vi "test Configure SLSC Switch Custom Device from Switches JSON.vi"(8 "error in (no error)":errorcluster, 11 "TestCase in":refnum<class "NI-SWITCH Scripting Unit Tests.lvclass">) -> (0 "error out":errorcluster, 3 "TestCase out":refnum<class "NI-SWITCH Scripting Unit Tests.lvclass">)   [LabVIEW 2017, in "NI-SWITCH Scripting Unit Tests.lvclass"]
uses:
  NI-SWITCH Scripting Unit Tests.lvclass
  <vilib>/addons/_JKI Toolkits/VI Tester/TestCase.llb/TestCase.lvclass
  NI-SWITCH Scripting.lvlib
  Shared/Endpoint Configuration Enum.ctl
  Shared/NI-SWITCH Shared.lvlib
  Shared/Endpoint Configuration Cluster.ctl
  Custom Device/Find All SLSC Switch Custom Devices.vi
  Shared/Routing and Faulting Hardware API/Routing and Faulting Hardware API.lvlib
  C:/Program Files (x86)/National Instruments/LabVIEW 2017/vi.lib/addons/_JKI Toolkits/VI Tester/TestCase.llb/TestCase.lvclass
panel:
  in  "Save?":bool
  out "Output Filename":string
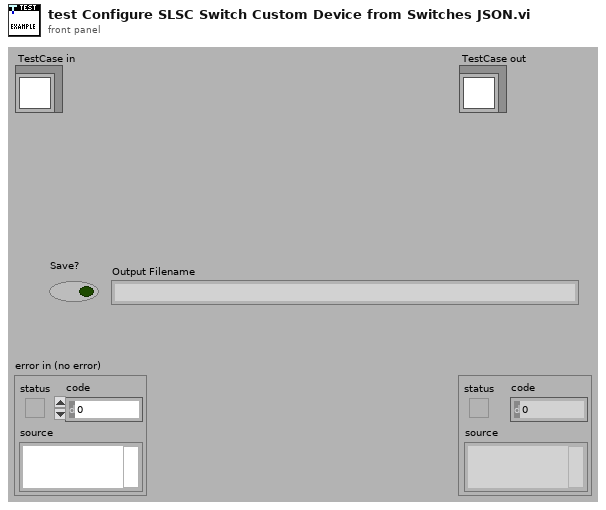
[diagram p1: front panel]
types:
  T1 = typedef "NI-SWITCH Shared.lvlib/Endpoint Configuration Cluster.ctl" = cluster{"Endpoint":string, "Configuration":T2}
  T2 = typedef "NI-SWITCH Shared.lvlib/Endpoint Configuration Enum.ctl" = enum16{"Load", "Source", "Configuration"}
  T3 = typedef "Custom Device API.lvlib/Custom Device Item Ref.ctl" = u64
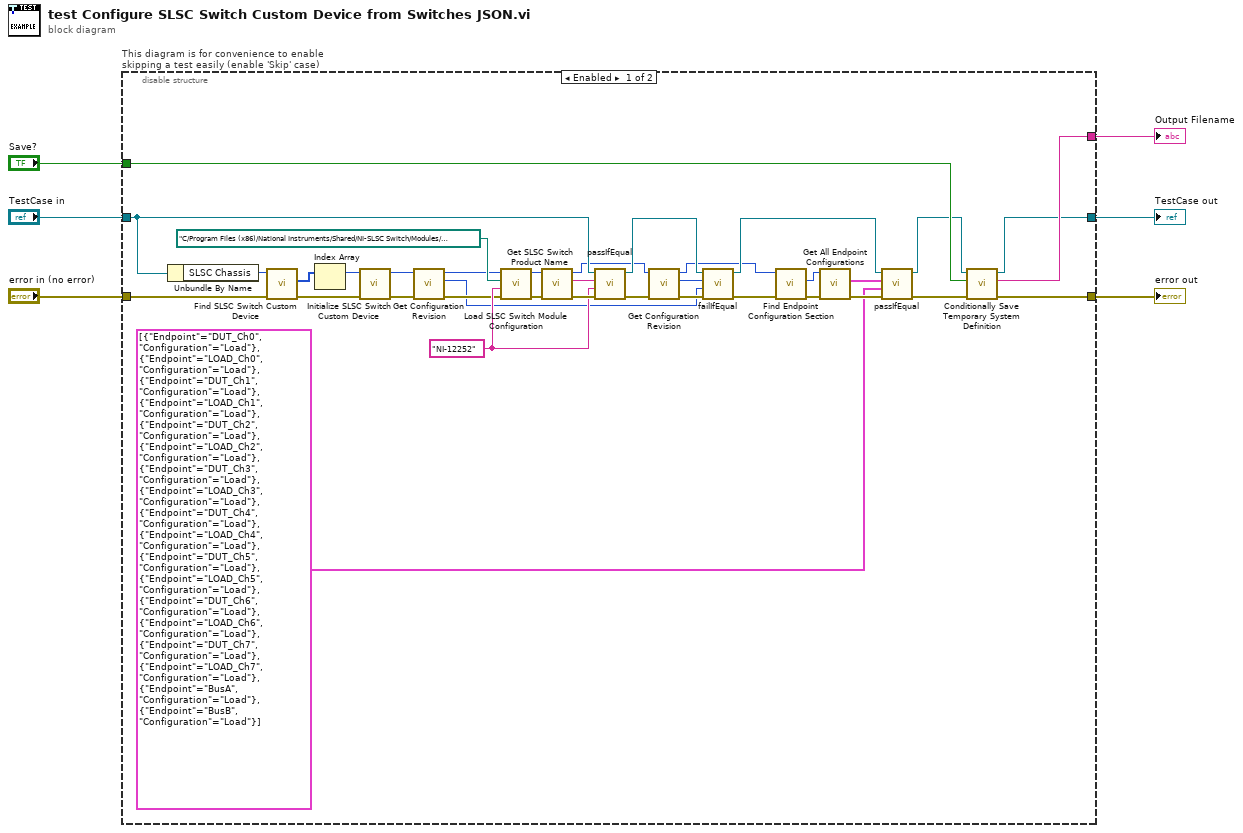
[diagram p0: block diagram]
diagram:
  n1 = disable-structure "This diagram is for convenience to enable skipping a test easily (enable 'Skip' case)" shown="Enabled" {
    disable-tunnel: "TestCase in" -> [w32 w46]
    disable-tunnel: [w40 w44] -> w3
    disable-tunnel: [w41 w45] -> w5
    disable-tunnel: "error in (no error)" -> [w36 w43]
    disable-tunnel: [w42 _] -> w2
    disable-tunnel: "Save?" -> [w39 _]
    frame Enabled {
      w20 = "NI-12252" ("Model")
      n2 = Unbundle By Name(w32) -> ("SLSC Chassis"=w37:u64)
      n3 = call-poly "Find SLSC Switch Custom Device.vi"("error in"=w36, "slsc chassis in"=w37) -> ("error out"=w34:errorcluster, "slsc switch custom devices"=w38:T3[])  [unwired: 7 in, 1 out]
      n4 = Index Array(array=w38) -> (element=w35:T3)  [unwired: 1 in]
      n5 = call "Initialize SLSC Switch Custom Device.vi"("error in"=w34, "slsc switch custom device in"=w35) -> ("error out"=w19:errorcluster, "slsc switch custom device out"=w17:T3)  [unwired: 7 in, 1 out]
      n6 = call "Get Configuration Revision.vi"("error in (no error)"=w19, "Hardware Ref in"=w17) -> ("error out"=w18:errorcluster, "Configuration Revision"=w10:u32, "Hardware Ref out"=w16:T3)  [unwired: 6 in, 1 out]
      n7 = call "Load SLSC Switch Module Configuration.vi"("error in"=w18, "product name"=w20, "switches json file"=path "C:/Program Files (x86)/National Instruments/Shared/NI-SLSC Switch/Modules/SLSC-12252-switches.json" ("switches JSON file"), "slsc switch custom device in"=w16) -> ("error out"=w21:errorcluster, "slsc switch custom device out"=w31:T3)  [unwired: 6 in]
      n8 = call "Get SLSC Switch Product Name.vi"("error in"=w21, "slsc switch custom device in"=w31) -> ("error out"=w30:errorcluster, "product name"=w29:string, "slsc switch custom device out"=w8:T3)  [unwired: 7 in]
      n9 = call-dynamic "passIfEqual.vi"("error in (no error)"=w30, "y"=w20, "x"=w29, "TestCase in"=w32) -> ("error out"=w13:errorcluster, "TestCase out"=w15:refnum<class "NI-SWITCH Scripting Unit Tests.lvclass">)  [unwired: 6 in]
      n10 = call "Get Configuration Revision.vi"("error in (no error)"=w13, "Hardware Ref in"=w8) -> ("error out"=w12:errorcluster, "Configuration Revision"=w11:u32, "Hardware Ref out"=w7:T3)  [unwired: 6 in, 1 out]
      n11 = call-dynamic "failIfEqual.vi"("error in (no error)"=w12, "y"=w10, "x"=w11, "TestCase in"=w15) -> ("error out"=w9:errorcluster, "TestCase out"=w14:refnum<class "NI-SWITCH Scripting Unit Tests.lvclass">)  [unwired: 6 in]
      n12 = call "Find Endpoint Configuration Section.vi"("error in"=w9, "slsc switch custom device in"=w7) -> ("error out"=w25:errorcluster, "endpoint configuration"=w24:T3)  [unwired: 7 in, 1 out]
      n13 = call "Get All Endpoint Configurations.vi"("error in"=w25, "endpoint configuration in"=w24) -> ("error out"=w28:errorcluster, "endpoint configurations"=w22:T1[])  [unwired: 7 in, 1 out]
      n14 = call-dynamic "passIfEqual.vi"("error in (no error)"=w28, "y"=T1[] [{"Endpoint"="DUT_Ch0", "Configuration"=enum."Load"}, {"Endpoint"="LOAD_Ch0", "Configuration"=enum."Load"}, {"Endpoint"="DUT_Ch1", "Configuration"=enum."Load"}, {"Endpoint"="LOAD_Ch1", "Configuration"=enum."Load"}, {"Endpoint"="DUT_Ch2", "Configuration"=enum."Load"}, {"Endpoint"="LOAD_Ch2", "Configuration"=enum."Load"}, {"Endpoint"="DUT_Ch3", "Configuration"=enum."Load"}, {"Endpoint"="LOAD_Ch3", "Configuration"=enum."Load"}, {"Endpoint"="DUT_Ch4", "Configuration"=enum."Load"}, {"Endpoint"="LOAD_Ch4", "Configuration"=enum."Load"}, {"Endpoint"="DUT_Ch5", "Configuration"=enum."Load"}, {"Endpoint"="LOAD_Ch5", "Configuration"=enum."Load"}, {"Endpoint"="DUT_Ch6", "Configuration"=enum."Load"}, {"Endpoint"="LOAD_Ch6", "Configuration"=enum."Load"}, {"Endpoint"="DUT_Ch7", "Configuration"=enum."Load"}, {"Endpoint"="LOAD_Ch7", "Configuration"=enum."Load"}, {"Endpoint"="BusA", "Configuration"=enum."Load"}, {"Endpoint"="BusB", "Configuration"=enum."Load"}] ("All Endpoint Configurations"), "x"=w22, "TestCase in"=w14) -> ("error out"=w27:errorcluster, "TestCase out"=w26:refnum<class "NI-SWITCH Scripting Unit Tests.lvclass">)  [unwired: 6 in]
      n15 = call "Conditionally Save Temporary System Definition.vi"("error in (no error)"=w27, "Save?"=w39, "Test Case"=w26) -> ("error out"=w41:errorcluster, "filename"=w42:string, "Test Case"=w40:refnum<class "NI-SWITCH Scripting Unit Tests.lvclass">)  [unwired: 6 in]
    }
    frame Disabled {
      # "skip test result while test is under development"
      n16 = call <vilib>:"skip.vi"("error in (no error)"=w43, "TestCase in"=w46) -> ("error out"=w45:errorcluster, "TestCase out"=w44:refnum<class "NI-SWITCH Scripting Unit Tests.lvclass">)  [unwired: 8 in]
    }
  }
  "error out" <- w5
  "TestCase out" <- w3
  "Output Filename" <- w2
